vi "DatabaseWithWebsite.vi"() -> ()   [LabVIEW 2018]
uses:
  <vilib>/drjdpowell/SQLite Library/SQL Statement/SQL Statement.lvclass/SQL Statement.ctl
  <vilib>/drjdpowell/SQLite Library/SQL Connection/Open (path).vi
  <vilib>/drjdpowell/SQLite Library/SQL Statement/Bind Text.vi
  <vilib>/drjdpowell/SQLite Library/SQL Connection/Open (string).vi
  <vilib>/drjdpowell/SQLite Library/SQL Statement/Step.vi
  <vilib>/AdvancedString/Path To Command Line String.vi
  <vilib>/drjdpowell/SQLite Library/SQL Connection/Execute SQL (No results).vi
  <vilib>/drjdpowell/SQLite Library/SQL Statement/Error Message.vi
  <vilib>/regexp/Match Regular Expression.xnode
  <vilib>/drjdpowell/SQLite Library/SQL Connection/Connection.lvclass
  <vilib>/drjdpowell/SQLite Library/SQLite.lvlib
  <vilib>/drjdpowell/SQLite Library/SQL Statement/SQL Statement.lvclass
  <vilib>/drjdpowell/SQLite Library/Transaction Helpers/Transaction.lvlib
  <vilib>/httpClient/LabVIEWHTTPClient.lvlib
panel:
  out "Description 2":string
  out "Part Number 2":string
  out "Serial Number 2":string
  in  "Database Delete":bool
  in  "Database Path":path
  in  "Create New DB":bool
  in  "Exit":bool
  in  "Database Saving Add In":bool
  in  "Retrieve From HTTP":bool
  in  "Serial Number":string
  in  "Location":string(combo)
  in  "WebServices":string(combo)
  in  "Oracle Host":string(combo)
  out "Description":string
  out "Part Number":string
  out "Serial Number":string
  out "Retrieve Info":string
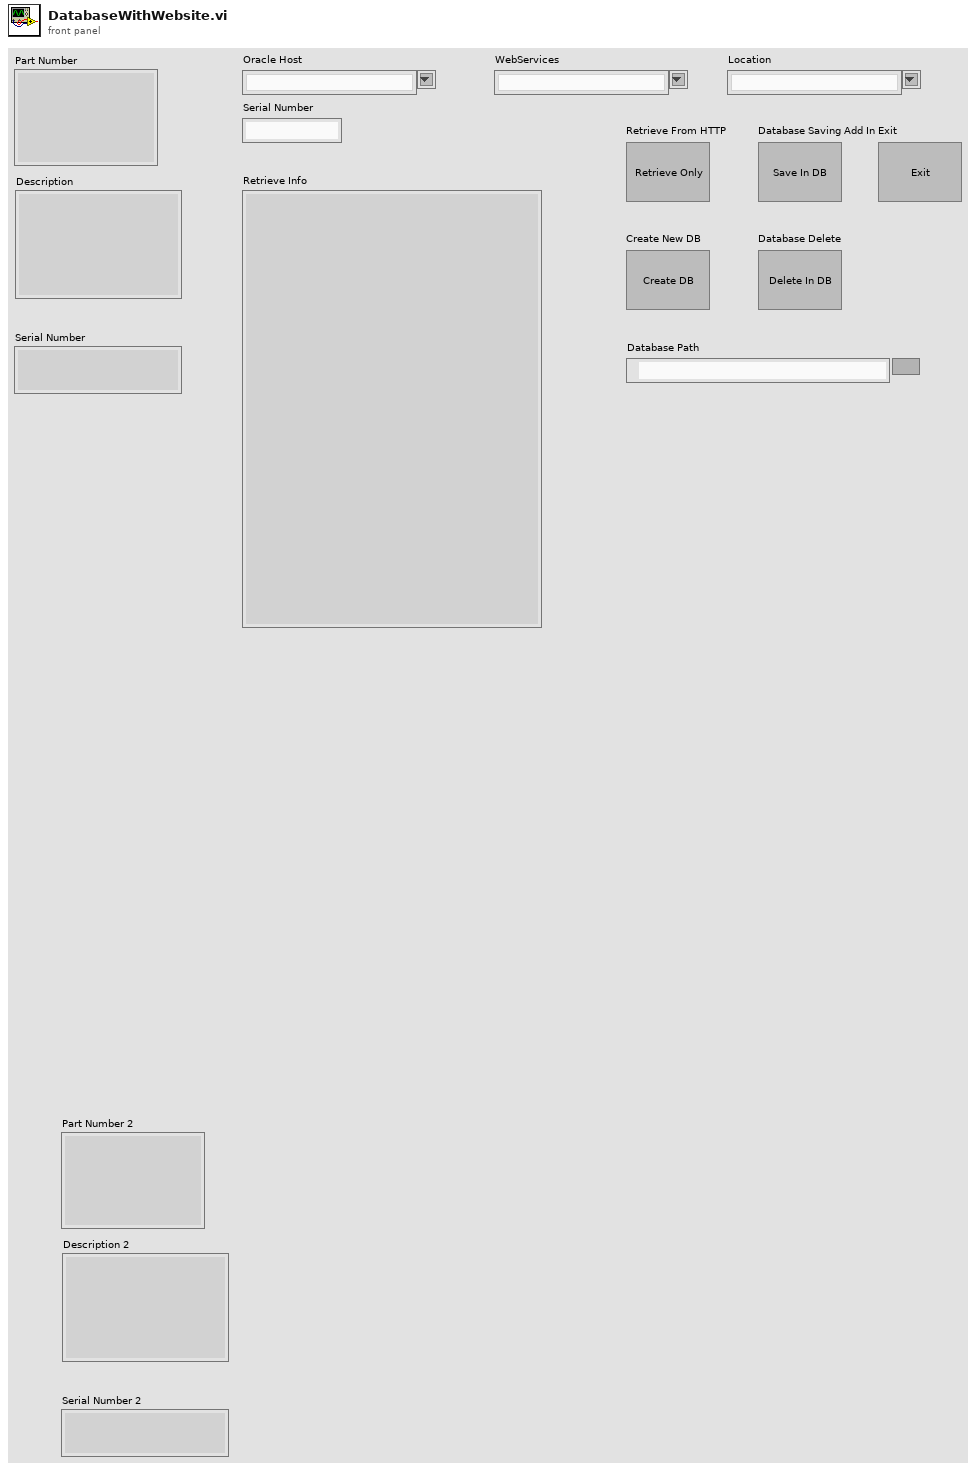
[diagram p1: front panel]
types:
  T1 = typedef "LabVIEWHTTPClient.lvlib/ClientHandle.ctl" = refnum<k1>
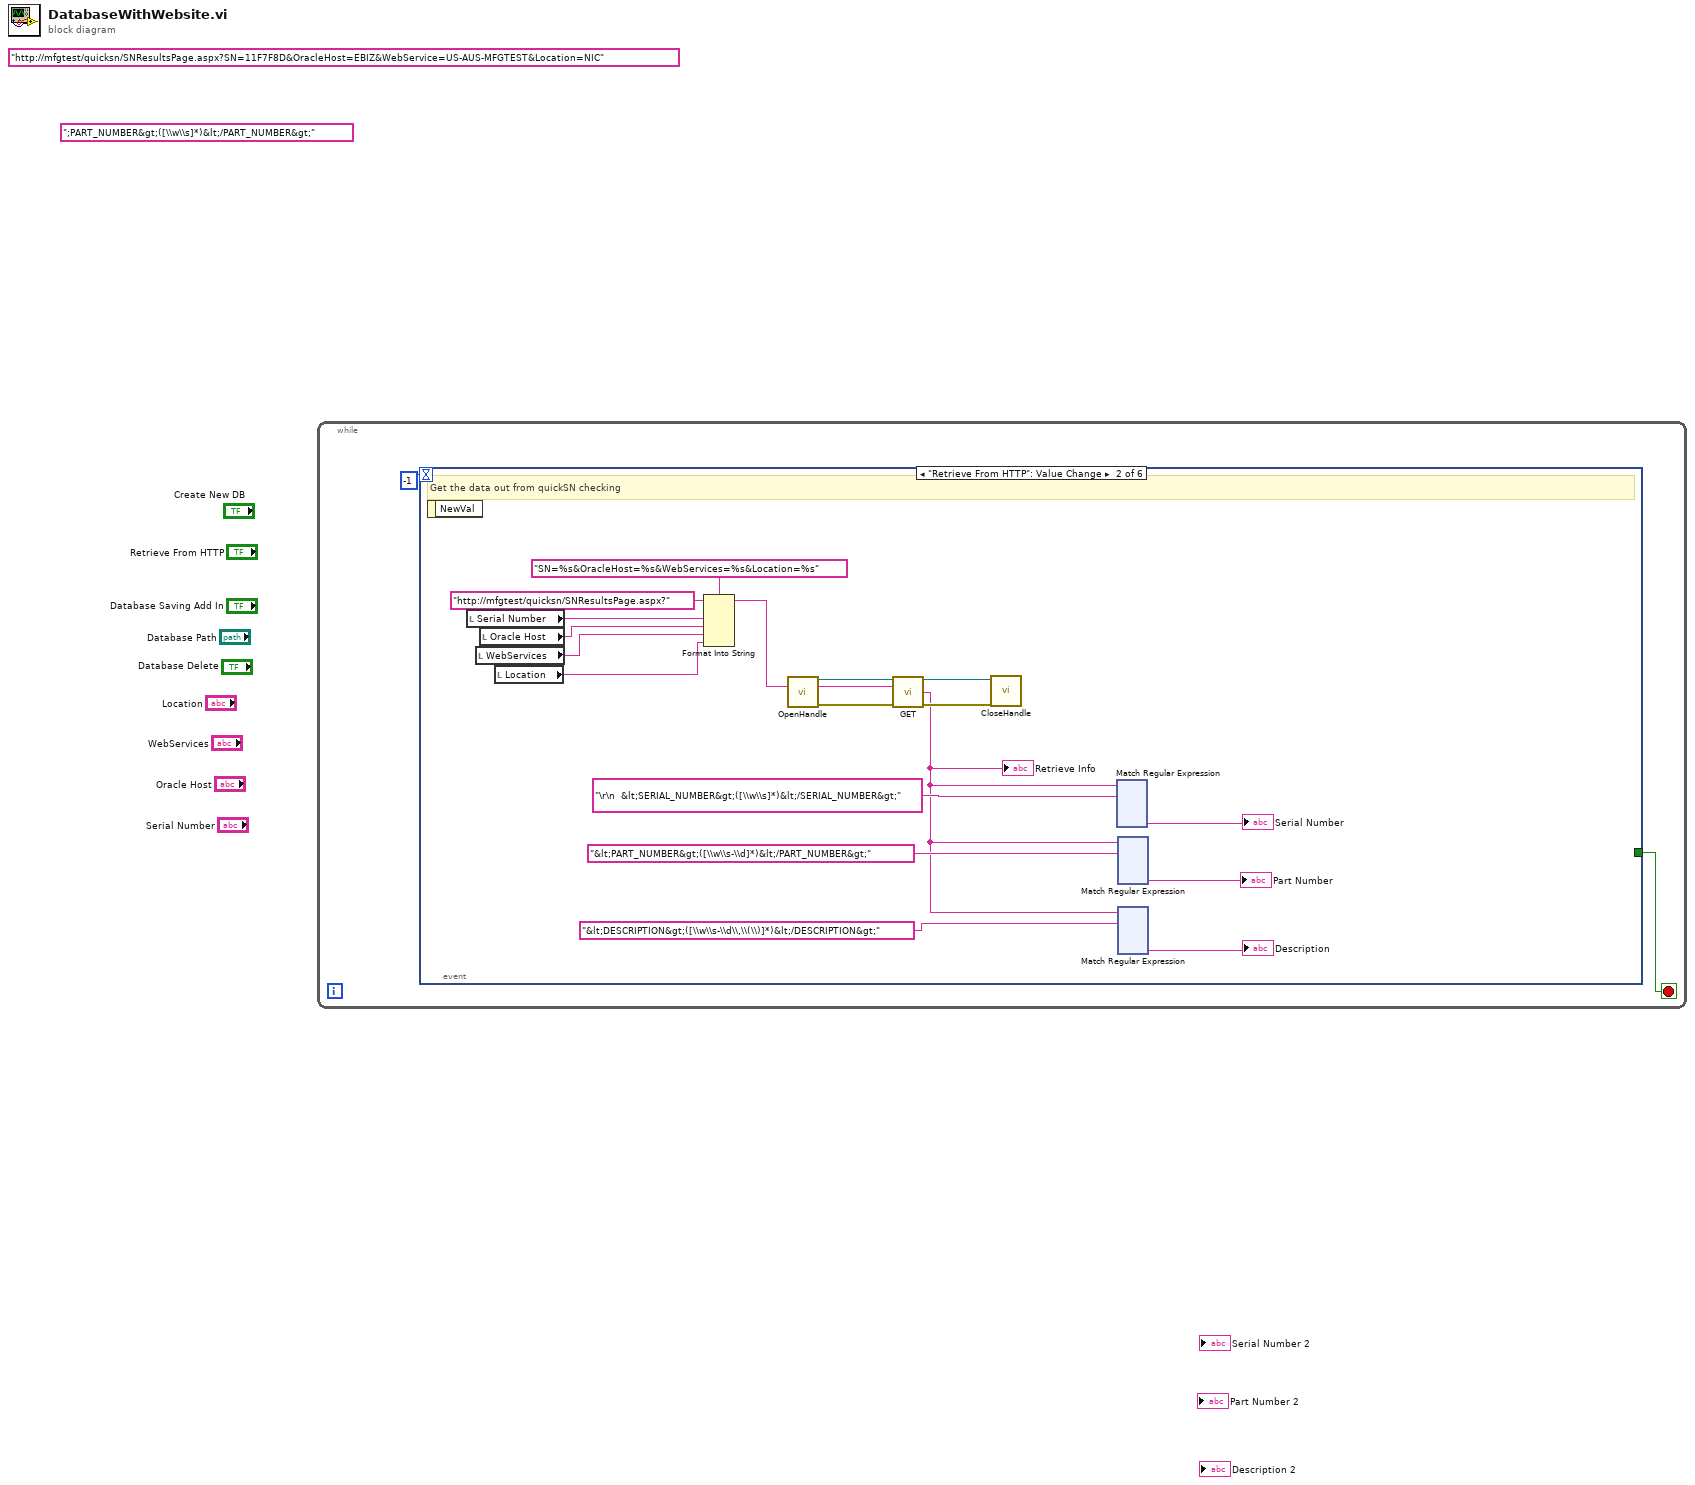
[diagram p0: block diagram]
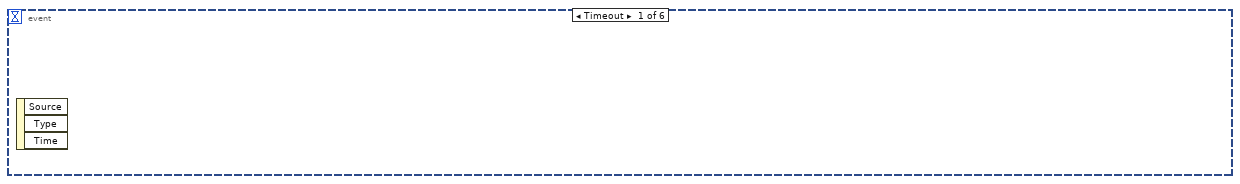
[diagram p2: hidden frame]
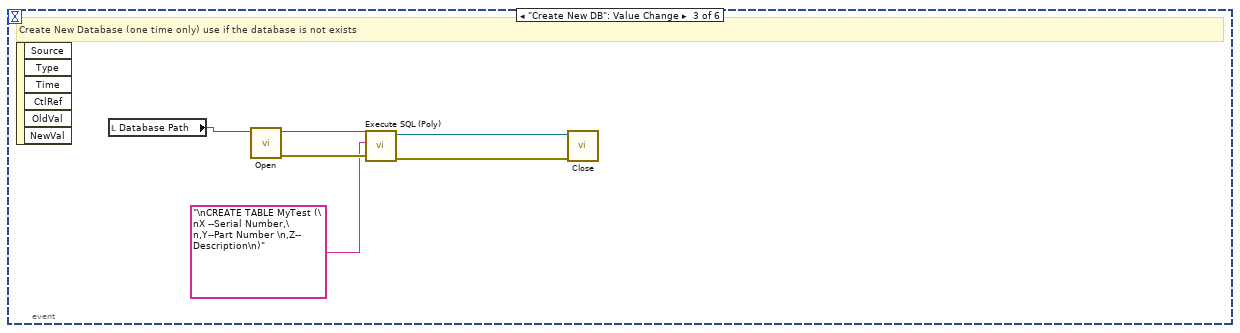
[diagram p3: hidden frame]
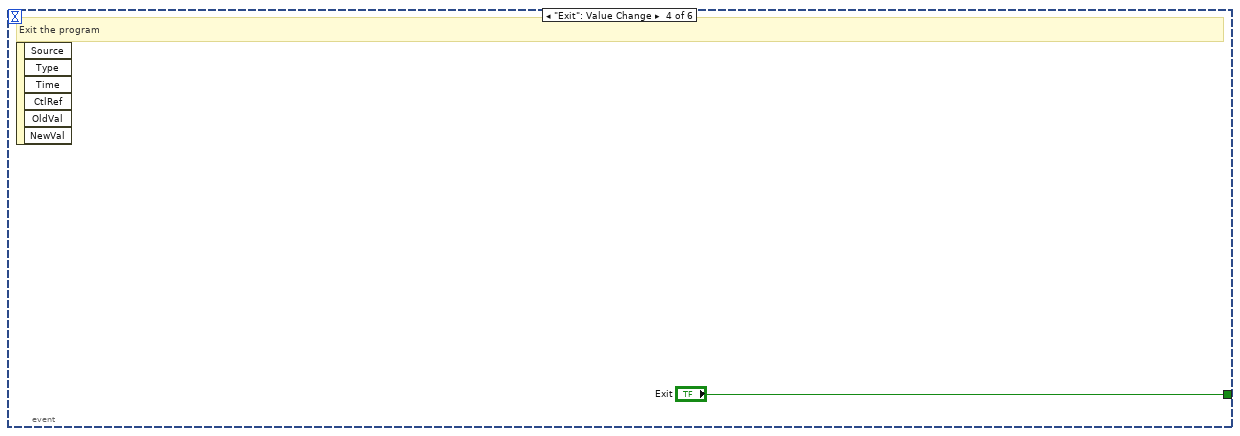
[diagram p4: hidden frame]
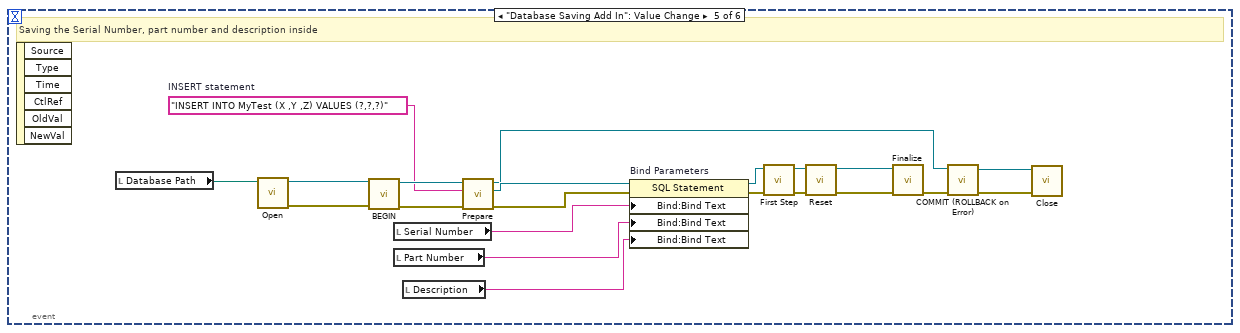
[diagram p5: hidden frame]
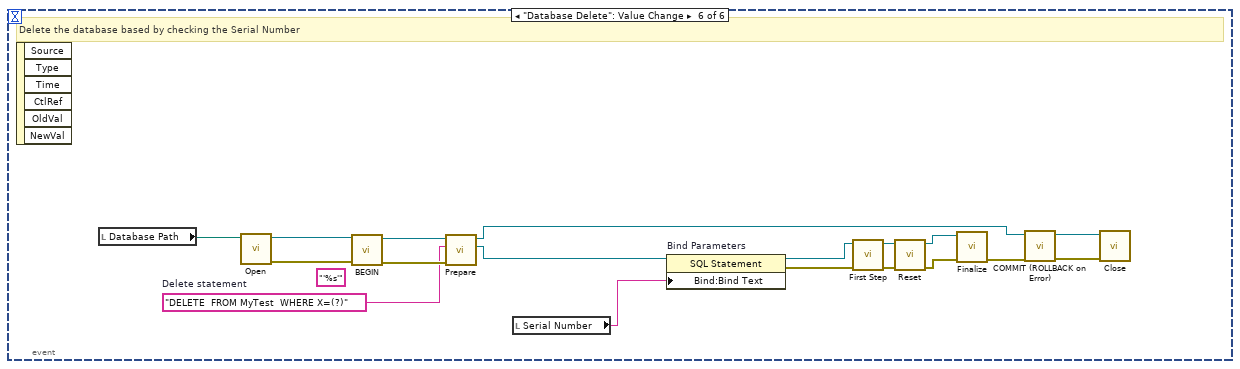
[diagram p6: hidden frame]
diagram:
  (unwired) ";PART_NUMBER&gt;([\\w\\s]*)&lt;/PART_NUMBER&gt;" ("regular expression")
  (unwired) "http://mfgtest/quicksn/SNResultsPage.aspx?SN=11F7F8D&OracleHost=EBIZ&WebService=US-AUS-MFGTEST&Location=NIC" ("url")
  n1 = while {
    stop <- w1 stop-if-true
    n2 = event shown="[1] \"Retrieve From HTTP\": Value Change" {
      selector: _ -> [_ _ _ _ _ _]
      dyn-events: _ -> [_ _ _ _ _ _]
      timeout: -1 -> [_ _ _ _ _ _]
      tunnel: [_ _ _ "Exit" _ _] -> w1
      event Timeout {
        n3 = event-data() -> ()  [unwired: 1 in, 3 out]
      }
      event "Retrieve From HTTP": Value Change {
        # "Get the data out from quickSN checking"
        n4 = event-data() -> ()  [unwired: 1 in, 1 out]
        n5 = local read "Serial Number"() -> (w14:string)
        n6 = local read "WebServices"() -> (w12:string)
        n7 = local read "Oracle Host"() -> (w13:string)
        n8 = local read "Location"() -> (w11:string)
        n9 = Format Into String(format string="SN=%s&OracleHost=%s&WebServices=%s&Location=%s", initial string="http://mfgtest/quicksn/SNResultsPage.aspx?", w14, w13, w12, w11) -> (resulting string=w10:string)  [unwired: 1 in, 1 out]
        n10 = call <vilib>:"OpenHandle.vi"() -> ("client handle out"=w20:T1, "error out"=w18:errorcluster)  [unwired: 14 in]
        n11 = call <vilib>:"GET.vi"("client handle"=w20, "url"=w10, "error in (no error)"=w18) -> ("client handle out"=w19:T1, "body"=w6:string, "error out"=w17:errorcluster)  [unwired: 9 in, 1 out]
        "Retrieve Info" <- w6
        n12 = call <vilib>:"CloseHandle.vi"("client handle"=w19, "error in (no error)"=w17) -> ()  [unwired: 13 in, 1 out]
        n13 = xnode "Match Regular Expression"("input string"=w6, "regular expression"="\r\n  &lt;SERIAL_NUMBER&gt;([\\w\\s]*)&lt;/SERIAL_NUMBER&gt;") -> ("submatch 1"=→"Serial Number":string)  [unwired: 4 in, 5 out]
        n14 = xnode "Match Regular Expression"("input string"=w6, "regular expression"="&lt;PART_NUMBER&gt;([\\w\\s-\\d]*)&lt;/PART_NUMBER&gt;") -> ("submatch 1"=→"Part Number":string)  [unwired: 4 in, 5 out]
        n15 = xnode "Match Regular Expression"("input string"=w6, "regular expression"="&lt;DESCRIPTION&gt;([\\w\\s-\\d\\,\\(\\)]*)&lt;/DESCRIPTION&gt;") -> ("submatch 1"=→"Description":string)  [unwired: 4 in, 5 out]
      }
      event "Create New DB": Value Change {
        # "Create New Database (one time only) use if the database is not exists"
        n16 = event-data() -> ()  [unwired: 1 in, 6 out]
        n17 = local read "Database Path"() -> (w369:path)
        n18 = call-poly <vilib>:"Open.vi"("db file"=w369) -> ("error out"=w371:errorcluster, "SQLite Connection"=w374:refnum<class "Connection.lvclass">)  [unwired: 9 in]
        n19 = call-poly <vilib>:"Execute SQL (Poly).vi"("error in (no error)"=w371, "SQL"="\nCREATE TABLE MyTest (\nX --Serial Number,\n,Y--Part Number \n,Z-- Description\n)", "SQLite Connection in"=w374) -> ("error out"=w372:errorcluster, "SQLite Connection"=w373:refnum<class "Connection.lvclass">)  [unwired: 7 in]
        n20 = call-dynamic "Close.vi"("error in (no error)"=w372, "SQLite Connection in"=w373) -> ()  [unwired: 9 in, 1 out]
      }
      event "Exit": Value Change {
        # "Exit the program"
        n21 = event-data() -> ()  [unwired: 1 in, 6 out]
      }
      event "Database Saving Add In": Value Change {
        w380 = "INSERT INTO MyTest (X ,Y ,Z) VALUES (?,?,?)"  # INSERT statement
        # "Saving the Serial Number, part number and description inside"
        n22 = event-data() -> ()  [unwired: 1 in, 6 out]
        n23 = local read "Database Path"() -> (w379:path)
        n24 = call-poly <vilib>:"Open.vi"("db file"=w379) -> ("error out"=w382:errorcluster, "SQLite Connection"=w396:refnum<class "Connection.lvclass">)  [unwired: 9 in]
        n25 = call <vilib>:"BEGIN.vi"("error in (no error)"=w382, "SQLite Connection in"=w396) -> ("error out"=w394:errorcluster, "SQLite Connection"=w395:refnum<class "Connection.lvclass">)  [unwired: 8 in]
        n26 = local read "Serial Number"() -> (w378:string)
        n27 = local read "Part Number"() -> (w376:string)
        n28 = local read "Description"() -> (w377:string)
        n29 = call <vilib>:"Prepare.vi"("error in (no error)"=w394, "SQL"=w380, "SQLite Connection in"=w395) -> ("error out"=w381:errorcluster, "SQL Statement"=w384:refnum<class "SQL Statement.lvclass">, "SQLite Connection"=w383:refnum<class "Connection.lvclass">)  [unwired: 4 in, 2 out]
        n30 = property on="Bind Parameters" class="SQL Statement"(reference=w384, error in=w381, "Bind:Bind Text"=w378, "Bind:Bind Text"=w376, "Bind:Bind Text"=w377) -> (reference out=w388:refnum<class "SQL Statement.lvclass">, error out=w389:errorcluster)
        n31 = call <vilib>:"First Step.vi"("error in (no error)"=w389, "SQL Statement in"=w388) -> ("error out"=w390:errorcluster, "SQL Statement"=w391:refnum<class "SQL Statement.lvclass">)  [unwired: 7 in, 1 out]
        n32 = call <vilib>:"Reset.vi"("error in (no error)"=w390, "SQL Statement in"=w391) -> ("error out"=w386:errorcluster, "SQL Statement"=w387:refnum<class "SQL Statement.lvclass">)  [unwired: 8 in]
        n33 = call <vilib>:"Finalize.vi"("error in (no error)"=w386, "SQL Statement in"=w387) -> ("error out"=w385:errorcluster)  [unwired: 9 in]
        n34 = call <vilib>:"COMMIT (ROLLBACK on Error).vi"("error in (no error)"=w385, "SQLite Connection in"=w383) -> ("error out"=w393:errorcluster, "SQLite Connection"=w392:refnum<class "Connection.lvclass">)  [unwired: 8 in]
        n35 = call-dynamic "Close.vi"("error in (no error)"=w393, "SQLite Connection in"=w392) -> ()  [unwired: 9 in, 1 out]
      }
      event "Database Delete": Value Change {
        (unwired) "'%s'" ("format string")
        w405 = "DELETE  FROM MyTest  WHERE X=(?)"  # Delete statement
        # "Delete the database based by checking the Serial Number"
        n36 = event-data() -> ()  [unwired: 1 in, 6 out]
        n37 = local read "Database Path"() -> (w410:path)
        n38 = call-poly <vilib>:"Open.vi"("db file"=w410) -> ("error out"=w411:errorcluster, "SQLite Connection"=w414:refnum<class "Connection.lvclass">)  [unwired: 9 in]
        n39 = call <vilib>:"BEGIN.vi"("error in (no error)"=w411, "SQLite Connection in"=w414) -> ("error out"=w412:errorcluster, "SQLite Connection"=w413:refnum<class "Connection.lvclass">)  [unwired: 8 in]
        n40 = call <vilib>:"Prepare.vi"("error in (no error)"=w412, "SQL"=w405, "SQLite Connection in"=w413) -> ("SQL Statement"=w404:refnum<class "SQL Statement.lvclass">, "SQLite Connection"=w401:refnum<class "Connection.lvclass">)  [unwired: 4 in, 3 out]
        n41 = local read "Serial Number"() -> (w398:string)
        n42 = property on="Bind Parameters" class="SQL Statement"(reference=w404, "Bind:Bind Text"=w398) -> (reference out=w406:refnum<class "SQL Statement.lvclass">, error out=w407:errorcluster)  [unwired: 1 in]
        n43 = call <vilib>:"First Step.vi"("error in (no error)"=w407, "SQL Statement in"=w406) -> ("error out"=w408:errorcluster, "SQL Statement"=w409:refnum<class "SQL Statement.lvclass">)  [unwired: 7 in, 1 out]
        n44 = call <vilib>:"Reset.vi"("error in (no error)"=w408, "SQL Statement in"=w409) -> ("error out"=w402:errorcluster, "SQL Statement"=w403:refnum<class "SQL Statement.lvclass">)  [unwired: 8 in]
        n45 = call <vilib>:"Finalize.vi"("error in (no error)"=w402, "SQL Statement in"=w403) -> ("error out"=w397:errorcluster)  [unwired: 9 in]
        n46 = call <vilib>:"COMMIT (ROLLBACK on Error).vi"("error in (no error)"=w397, "SQLite Connection in"=w401) -> ("error out"=w399:errorcluster, "SQLite Connection"=w400:refnum<class "Connection.lvclass">)  [unwired: 8 in]
        n47 = call-dynamic "Close.vi"("error in (no error)"=w399, "SQLite Connection in"=w400) -> ()  [unwired: 9 in, 1 out]
      }
    }
  }
